vi "TwTpsGetActiveFilament.vi"(0 "error in (no error)":errorcluster) -> (1 "error out":errorcluster, 2 "activeFilament":i32)   [LabVIEW 2009]
uses:
  TofDaqDll.dll
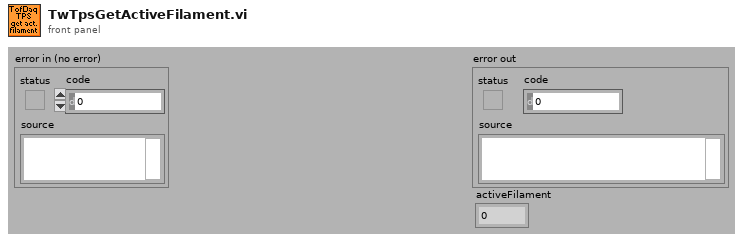
[diagram p1: front panel]
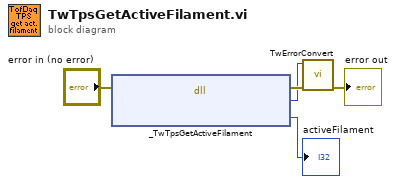
[diagram p0: block diagram]
diagram:
  n1 = dll-call lib="C:/src/TofDaq/APIandWrappers/LabView/TofDaqDll/TofDaqDll.dll" fn="_TwTpsGetActiveFilament"(error in="error in (no error)") -> (error out=w4:errorcluster, "TwRetVal"=w2:i32, "activeFilament"=→"activeFilament":i32)  [unwired: 3 in, 1 out]
  n2 = call "TwErrorConvert.vi"("error in (no error)"=w4, "error code"=w2) -> ("error out"=→"error out":errorcluster)  [unwired: 9 out]
